vi "ToggleState.vi"(0 "reference in":refnum<class "Security.lvclass">, 5 "Error In":errorcluster) -> (14 "reference out":refnum<class "Security.lvclass">, 19 "Error Out":errorcluster)   [LabVIEW 2024, in "Security.lvclass"]
doc: "Toggles current state property."
uses:
  Security.lvclass
  Security.lvclass/Security.ctl
panel:
  # "Connector Pane"
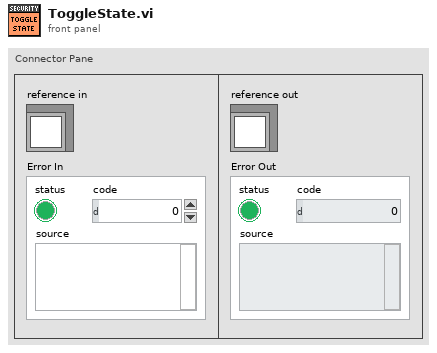
[diagram p1: front panel]
types:
  T1 = typedef "Security.lvclass/ObjectAttributes.ctl" = cluster{"State":bool, "Security Mode":T2}
  T2 = typedef "SecuritySystem.lvclass/Security Mode.ctl" = enum16{"Aggresive", "Defensive", "Balanced"}
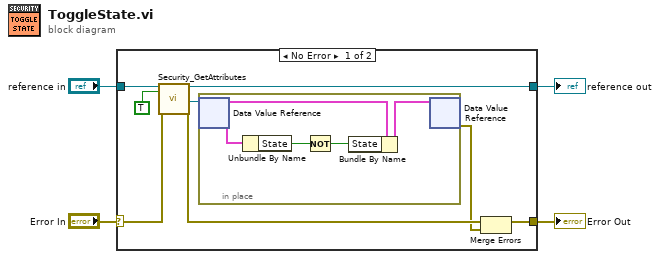
[diagram p0: block diagram]
diagram:
  n1 = case shown="No Error" "Error In" {
    selector: "Error In" -> [w11 w18]
    tunnel: [w9 w18] -> w3
    tunnel: [w10 w17] -> w1
    tunnel: "reference in" -> [w12 w17]
    frame No Error {
      n2 = call "Security_GetAttributes.vi"("reference in"=w12, "OnlyGetDvrReference(False)"=TRUE, "Error In"=w11) -> ("reference out"=w10:refnum<class "Security.lvclass">, "DataRef"=w8:refnum<data-value>, "Error Out"=w6:errorcluster)  [unwired: 13 in, 1 out]
      n3 = in-place {
        n4 = in-place-dvr #1(w8) -> (w15:T1)  [unwired: 1 out]
        n5 = Unbundle By Name(w15) -> ("State"=w14:bool)
        n6 = Not(x=w14) -> (.not. x?=w13:bool)
        n7 = Bundle By Name(cluster=w15, "State"=w13) -> (w16:T1)
        n8 = in-place-dvr #1(w16) -> (w5:errorcluster)  [unwired: 1 out]
      }
      n9 = Merge Errors(w6, w5) -> (w9:errorcluster)
    }
    frame Error {
    }
  }
  "Error Out" <- w3
  "reference out" <- w1
